vi "HRR-Error.vi"(8 "Status":u8, 10 "Nvezes":i32, 11 "error in (no error)":errorcluster) -> (3 "error out":errorcluster)   [LabVIEW 2019]
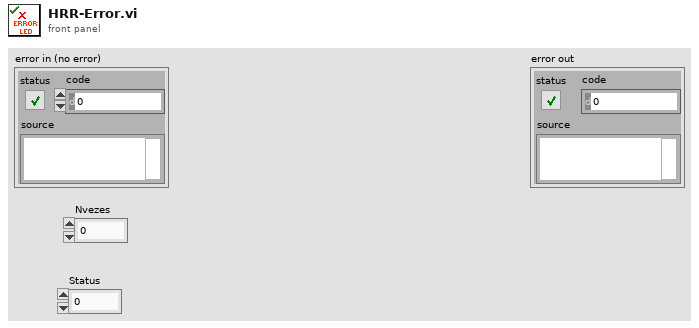
[diagram p1: front panel]
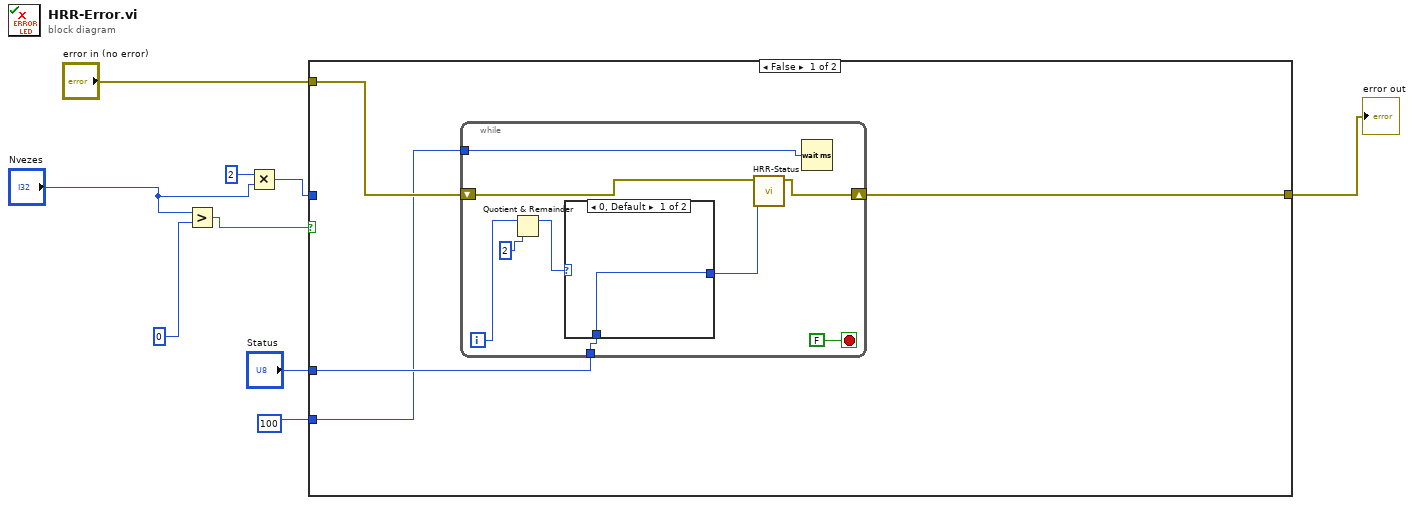
[diagram p0: block diagram]
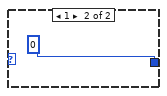
[diagram p2: hidden frame]
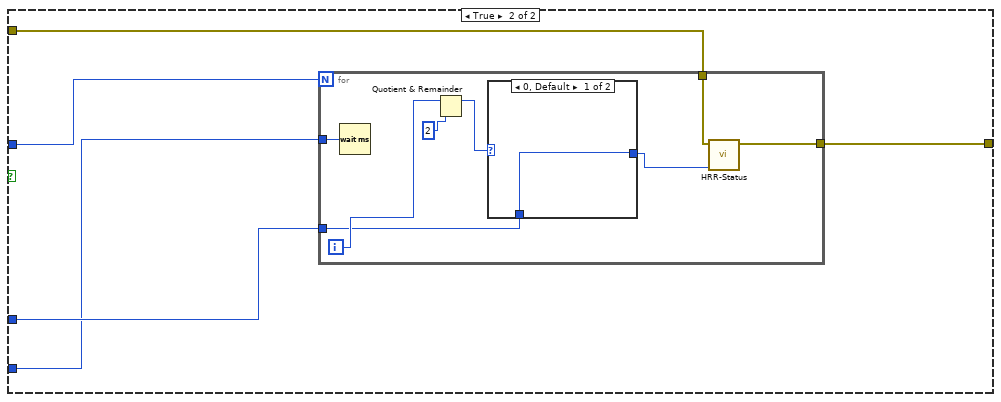
[diagram p3: hidden frame]
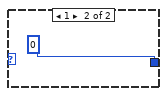
[diagram p4: hidden frame]
diagram:
  n1 = Greater?(x="Nvezes", y=0) -> (0:w6:bool)
  n2 = Multiply(x=2, y="Nvezes") -> (x*y=w2:i32)
  n3 = case shown="False" w6 {
    tunnel: "error in (no error)" -> [w13 w29]
    tunnel: [w12 w28] -> w8
    tunnel: w2 -> [_ w27]
    tunnel: "Status" -> [w11 w26]
    tunnel: u32 100 -> [w10 w25]
    frame False {
      n4 = while {
        shift-right: [w21] -> w12
        shift-left: w13 -> [w22]
        tunnel: w11 -> [w16]
        tunnel: w10 -> [w20]
        i -> [w19]
        stop <- FALSE stop-if-true
        n5 = Quotient & Remainder(x=w19, y=2) -> (x-y*floor(x/y)=w17:i32)  [unwired: 1 out]
        n6 = case shown="0, Default" w17 {
          tunnel: w16 -> [w23 _]
          tunnel: [w23 u8 0] -> w15
          frame 0, Default {
          }
          frame 1 {
          }
        }
        n7 = call "HRR-Status.vi"("Status (U4)"=w15, "error in (no error)"=w22) -> ("error out"=w21:errorcluster)  [unwired: 9 in]
        n8 = Wait (ms)(milliseconds to wait=w20) -> ()  [unwired: 1 out]
      }
    }
    frame True {
      n9 = for {
        N: w27 -> [_]
        tunnel: w29 -> [w37]
        tunnel: [w36] -> w28
        tunnel: w26 -> [w31]
        tunnel: w25 -> [w35]
        i -> [w32]
        n10 = Wait (ms)(milliseconds to wait=w35) -> ()  [unwired: 1 out]
        n11 = Quotient & Remainder(x=w32, y=2) -> (x-y*floor(x/y)=w33:i32)  [unwired: 1 out]
        n12 = case shown="0, Default" w33 {
          tunnel: w31 -> [w38 _]
          tunnel: [w38 u8 0] -> w30
          frame 0, Default {
          }
          frame 1 {
          }
        }
        n13 = call "HRR-Status.vi"("Status (U4)"=w30, "error in (no error)"=w37) -> ("error out"=w36:errorcluster)  [unwired: 9 in]
      }
    }
  }
  "error out" <- w8
